vi "Release Brake.vi"(8 "error in (no error)":errorcluster, 11 "Elevator in":refnum<class "Elevator.lvclass">) -> (0 "error out":errorcluster, 3 "Elevator out":refnum<class "Elevator.lvclass">)   [LabVIEW 2014, in "Elevator.lvlib" / "Elevator.lvclass"]
uses:
  Elevator.lvclass
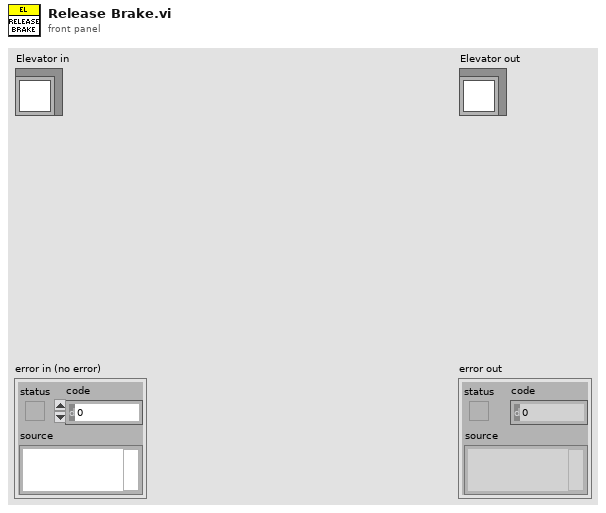
[diagram p1: front panel]
types:
  T1 = enum16{"Critical", "Error", "Warning", "Informational", "Debug"}
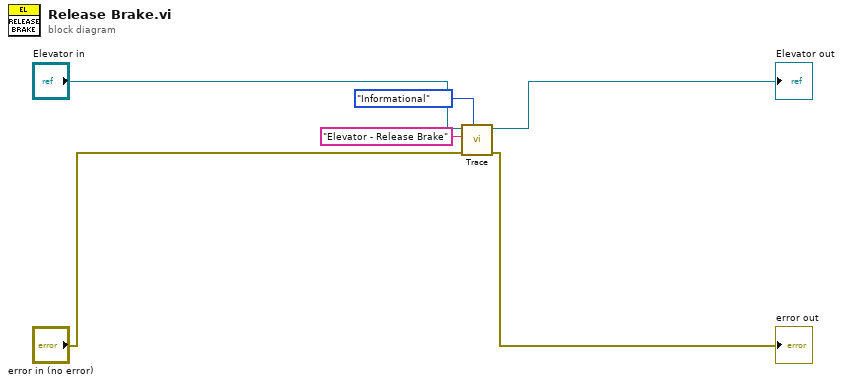
[diagram p0: block diagram]
diagram:
  n1 = call-dynamic "Trace.vi"("Trace Level"=T1."Informational", "error in (no error)"="error in (no error)", "System Action"="Elevator - Release Brake", "System Actor in"="Elevator in") -> ("error out"=→"error out":errorcluster, "System Actor out"=→"Elevator out":refnum<class "Elevator.lvclass">)  [unwired: 6 in]
